vi "Delete SFTP Refnum.vi"(8 "error in (no error)":errorcluster, 11 "sftp":T1) -> (0 "error out":errorcluster, 3 "LIBSSH2_SFTP*":u64)   [LabVIEW 2013, in "libssh2.lvlib"]
doc: "Delete <B>sftp</B> and return associated <B>LIBSSH2_SFTP*</B>."
uses:
  libssh2.lvlib
  SFTP Refnum.ctl
  SFTP Refnum Data.ctl
  Session Refnum.ctl
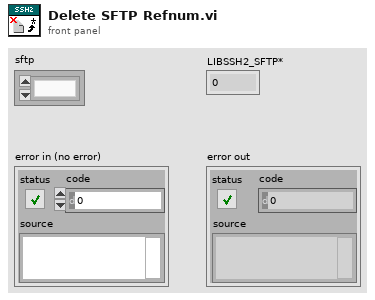
[diagram p1: front panel]
types:
  T1 = typedef "libssh2.lvlib/SFTP Refnum.ctl" = refnum<k1>
  T2 = typedef "libssh2.lvlib/SFTP Refnum Data.ctl" = cluster{"LIBSSH2_SFTP*":u64, "session":T3}
  T3 = typedef "libssh2.lvlib/Session Refnum.ctl" = refnum<k1>
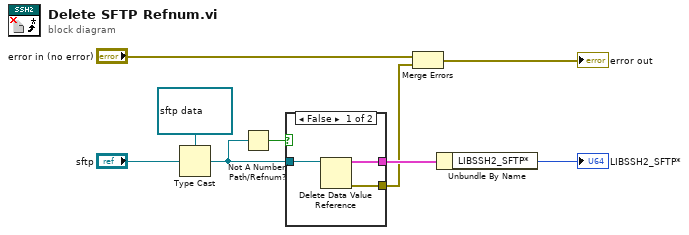
[diagram p0: block diagram]
diagram:
  n1 = Type Cast(type=refnum<data-value> refnum ("data value reference"), x="sftp") -> (*(type *) &x=w5:refnum<data-value>)
  n2 = Not A Number/Path/Refnum?(number/path/refnum=w5) -> (NaN/Path/Refnum?=w4:bool)
  n3 = case shown="False" w4 {
    tunnel: [w12 _] -> w7
    tunnel: [w11 _] -> w6
    tunnel: w5 -> [w10 _]
    frame False {
      n4 = Delete Data Value Reference(data value reference=w10) -> (data value=w12:T2, error out=w11:errorcluster)  [unwired: 1 in]
    }
    frame True {
    }
  }
  n5 = Merge Errors("error in (no error)", w6) -> (→"error out":errorcluster)
  n6 = Unbundle By Name(w7) -> ("LIBSSH2_SFTP*"=→"LIBSSH2_SFTP*":u64)
